vi "Colorify.vi"(8 "Front Panel":refnum<vi>, 9 "String 2":refnum<vi>, 11 "String":string) -> ()   [LabVIEW 2020]
panel:
  out "End":i32
  out "Start":i32
  out "Occurances":i32
  out "Line Number":i32
  out "Good?":bool
  out "Before Error":i32
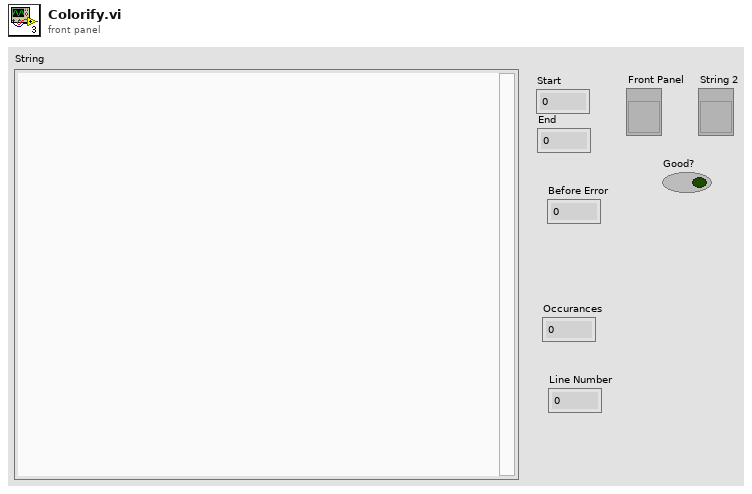
[diagram p1: front panel]
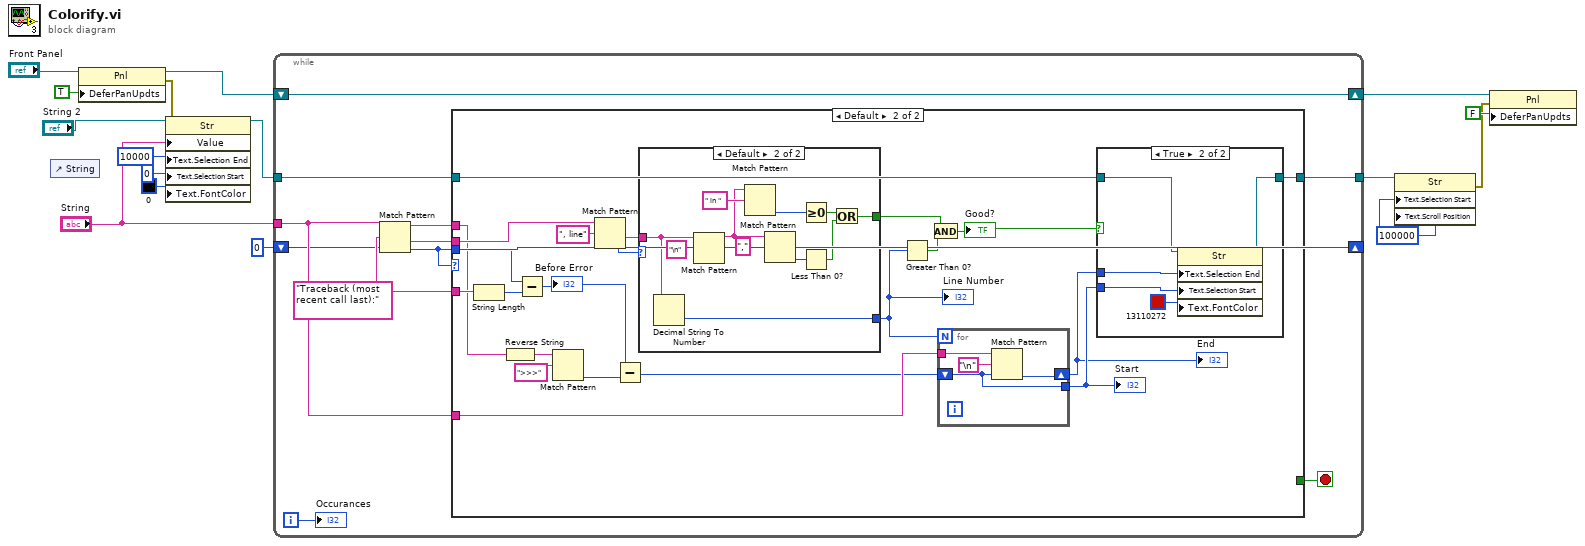
[diagram p0: block diagram]
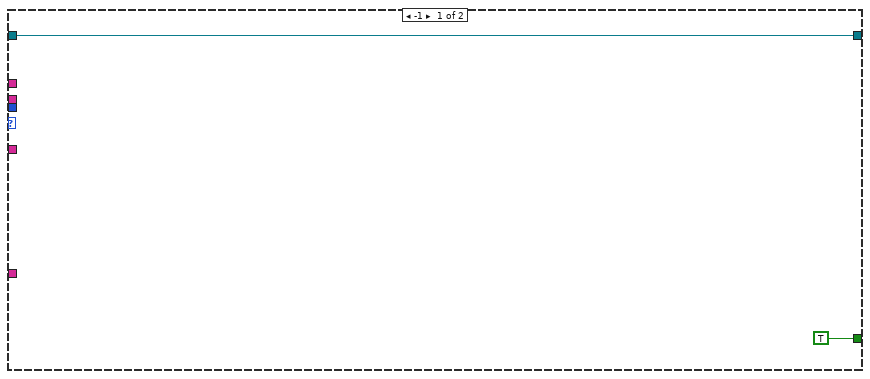
[diagram p2: hidden frame]
diagram:
  w6 = u32 100000 ("Text.Selection:Start")
  n1 = control-ref of="String"() -> ()  [unwired: 1 out]
  n2 = property class="Pnl"(reference="Front Panel", "DeferPanUpdts"=TRUE ("Defer Panel Updates")) -> (reference out=w13:refnum<vi>, error out=w1:errorcluster)  [unwired: 1 in]
  n3 = property on="Property Node" class="Str"(reference="String 2", error in=w1, "Value"="String", "Text.Selection End"=u32 10000 ("Text.Selection:End"), "Text.Selection Start"=u32 0 ("Text.Selection:Start"), "Text.FontColor"=u32 0 ("Text.Font:Color")) -> (reference out=w4:refnum<vi>)  [unwired: 1 out]
  n4 = while {
    tunnel: "String" -> [w24]
    shift-right: [w22] -> w14
    shift-left: w13 -> [w22]
    shift-right: [w21] -> _
    shift-left: 0 ("offset (0)") -> [w23]
    tunnel: w4 -> [w19]
    tunnel: [w17] -> w3
    i -> [w18]
    stop <- w20 stop-if-true
    w27 = "Traceback (most recent call last):"
    n5 = Match Pattern(string=w24, regular expression=w27, offset (0)=w23) -> (before substring=w25:string, after substring=w26:string, offset past match=w21:i32)  [unwired: 1 out]
    n6 = case shown="Default" w21 {
      tunnel: w27 -> [_ w50]
      tunnel: w26 -> [_ w43]
      tunnel: w25 -> [_ w40]
      tunnel: w24 -> [_ w39]
      tunnel: w21 -> [_ w35]
      tunnel: [TRUE _] -> w20
      tunnel: w19 -> [w28 w33]
      tunnel: [w28 w30] -> w17
      frame -1 {
      }
      frame Default {
        n7 = String Length(string=w50) -> (length=w51:i32)
        n8 = Reverse String(1:w40) -> (0:w42:string)
        n9 = Subtract(x=w35, y=w51) -> (x-y=w34:i32)
        "Before Error" <- w34
        n10 = Match Pattern(string=w42, regular expression=">>>") -> (offset past match=w32:i32)  [unwired: 1 in, 3 out]
        n11 = Match Pattern(string=w43, regular expression=", line") -> (after substring=w48:string, offset past match=w45:i32)  [unwired: 1 in, 2 out]
        n12 = Subtract(x=w34, y=w32) -> (x-y=w31:i32)
        n13 = case shown="Default" w45 {
          tunnel: w48 -> [_ w64]
          tunnel: [_ w63] -> w46
          tunnel: [_ w62] -> w37
          frame -1 {
          }
          frame Default {
            n14 = Decimal String To Number(string=w64) -> (number=w62:i32)  [unwired: 2 in, 1 out]
            n15 = Match Pattern(string=w64, regular expression="\n") -> (before substring=w68:string)  [unwired: 1 in, 3 out]
            n16 = Match Pattern(string=w68, regular expression=" in ") -> (offset past match=w69:i32)  [unwired: 1 in, 3 out]
            n17 = Match Pattern(string=w68, regular expression=",") -> (offset past match=w67:i32)  [unwired: 1 in, 3 out]
            n18 = Greater Or Equal To 0?(x=w69) -> (x >= 0?=w65:bool)
            n19 = Less Than 0?(x=w67) -> (x < 0?=w66:bool)
            n20 = Or(x=w65, y=w66) -> (x .or. y?=w63:bool)
          }
        }
        "Line Number" <- w37
        n21 = Greater Than 0?(x=w37) -> (x > 0?=w47:bool)
        n22 = And(x=w46, y=w47) -> (x .and. y?=w44:bool)
        "Good?" <- w44
        n23 = for {
          N: w37 -> [_]
          tunnel: w39 -> [w55]
          shift-right: [w53] -> w36
          shift-left: w31 -> [w52]
          tunnel: [w52] -> w38
          n24 = Match Pattern(string=w55, regular expression="\n", offset (0)=w52) -> (offset past match=w53:i32)  [unwired: 3 out]
        }
        "Start" <- w38
        "End" <- w36
        n25 = case shown="True" w44 {
          tunnel: w36 -> [_ w57]
          tunnel: w38 -> [_ w58]
          tunnel: w33 -> [w56 w60]
          tunnel: [w56 w59] -> w30
          frame False {
          }
          frame True {
            n26 = property on="Property Node" class="Str"(reference=w60, "Text.Selection End"=w57, "Text.Selection Start"=w58, "Text.FontColor"=u32 13110272) -> (reference out=w59:refnum<vi>)  [unwired: 1 in, 1 out]
          }
        }
      }
    }
    "Occurances" <- w18
  }
  n27 = property on="Property Node" class="Str"(reference=w3, "Text.Selection Start"=w6, "Text.Scroll Position"=w6) -> (error out=w5:errorcluster)  [unwired: 1 in, 1 out]
  n28 = property class="Pnl"(reference=w14, error in=w5, "DeferPanUpdts"=FALSE ("Defer Panel Updates")) -> ()  [unwired: 2 out]
